vi "checkBoard.vi"(1 "column":i32, 2 "row":i32, 3 "white":bool[][](array[boolean]), 4 "black":bool[][](array[boolean])) -> (0 "element":bool)   [LabVIEW 2014]
panel:
  out "mergeBoard":bool[][](array[boolean])
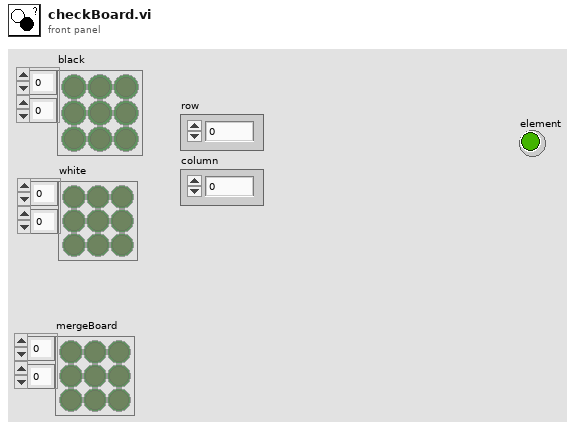
[diagram p1: front panel]
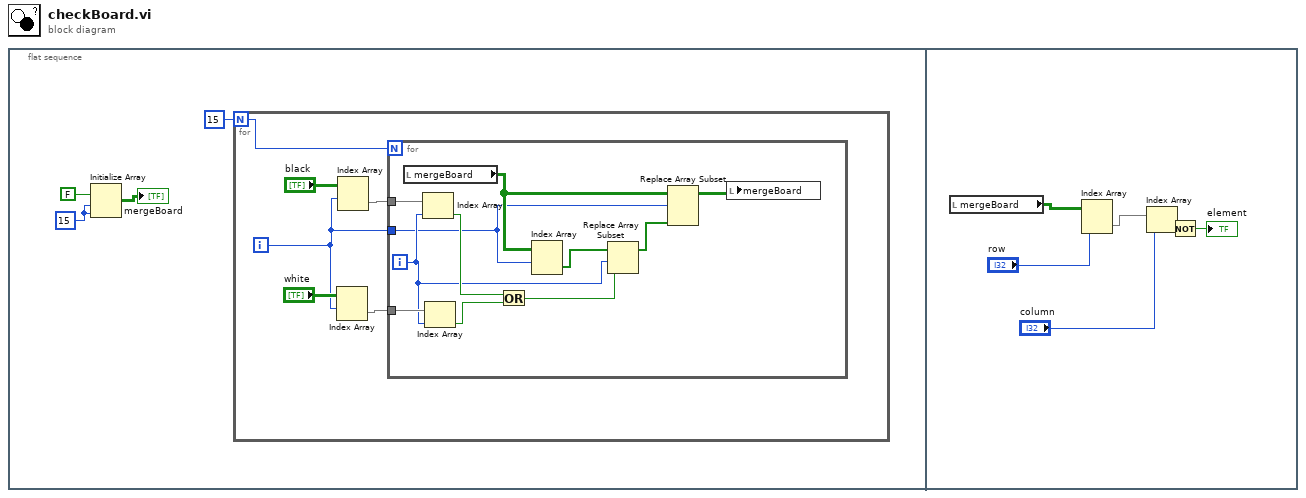
[diagram p0: block diagram]
diagram:
  n1 = flat-sequence {
    frame #0 {
      w1 = 15
      n2 = Initialize Array(FALSE, w1, w1) -> (→"mergeBoard":bool[][])
      n3 = for {
        N: 15 -> [w7]
        i -> [w5]
        n4 = Index Array(array="white", index (row)=w5) -> (element=w9:bool[])  [unwired: 1 in]
        n5 = Index Array(array="black", index (row)=w5) -> (element=w8:bool[])  [unwired: 1 in]
        n6 = for {
          N: w7 -> [_]
          tunnel: w9 -> [w20]
          tunnel: w8 -> [w21]
          tunnel: w5 -> [w13]
          i -> [w16]
          n7 = local read "mergeBoard"() -> (w14:bool[][])
          n8 = Index Array(array=w21, index=w16) -> (element=w19:bool)
          n9 = Index Array(array=w20, index=w16) -> (element=w18:bool)
          n10 = Or(x=w19, y=w18) -> (x .or. y?=w15:bool)
          n11 = Index Array(array=w14, index (row)=w13) -> (element=w17:bool[])  [unwired: 1 in]
          n12 = Replace Array Subset(array=w17, new element=w15, index=w16) -> (w11:bool[])
          n13 = Replace Array Subset(array=w14, new element=w11, index (row)=w13) -> (w12:bool[][])  [unwired: 1 in]
          n14 = local write "mergeBoard"(w12) -> ()
        }
      }
    }
    frame #1 {
      n15 = local read "mergeBoard"() -> (w27:bool[][])
      n16 = Index Array(array=w27, index (row)="row") -> (element=w25:bool[])  [unwired: 1 in]
      n17 = Index Array(array=w25, index="column") -> (element=w23:bool)
      n18 = Not(x=w23) -> (.not. x?=→"element":bool)
    }
  }
